vi "Engine - PFI - EGR Actuation Host.vi"() -> ()   [LabVIEW 2015, in "ECS-Host.lvlib"]
uses:
  ECS-Host.lvlib
  <vilib>/addons/Software Calibration Management/XControls/TBL1D.xctl
panel:
  in  "EGRPWM_E":bool
  in  "EGRPWMFreq":sgl caption="[Hz]"
  out "EGRPsnStp":sgl caption="[%Open]"
  out "EGRDutyCyc_TblOut":sgl caption="[%]"
  out "EGRDutyCyc_Des":sgl caption="[%]"
  in  "EGRDutyCyc_Tbl":cluster{"X":sgl[], "Y":sgl[]}(xcontrol)
  in  "EGRDutyCyc_ManE":bool
  in  "EGRDutyCyc_Man":sgl caption="[%]"
  in  "EGRDutyCyc_Min":sgl caption="[%]"
  in  "EGRDutyCyc_Max":sgl caption="[%]"
  # "EGR Actuator"
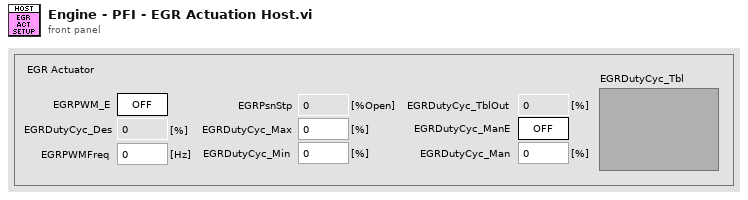
[diagram p1: front panel]
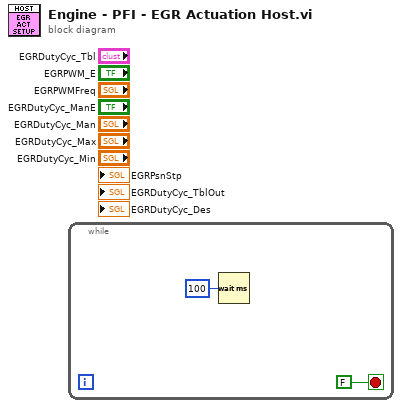
[diagram p0: block diagram]
diagram:
  n1 = while {
    stop <- FALSE stop-if-true
    n2 = Wait (ms)(milliseconds to wait=u32 100) -> ()  [unwired: 1 out]
  }
